vi "Flash Finish Stream.vi"(8 "error in (no error)":errorcluster, 11 "Orca-Flash 4.0 V2 in":refnum<class "Orca-Flash 4.0 V2.lvclass">) -> (0 "error out":errorcluster, 3 "Orca-Flash 4.0 V2 out":refnum<class "Orca-Flash 4.0 V2.lvclass">)   [LabVIEW 2017, in "Orca-Flash 4.0 V2.lvlib" / "Orca-Flash 4.0 V2.lvclass"]
uses:
  Orca-Flash 4.0 V2.lvclass
  C:/LVDEV/branch3/Flash Gordon v0.6.1b/Hardware/Camera/Camera.lvclass
  Orca-Flash 4.0 V2.lvclass/Orca-Flash 4.0 V2.ctl
  Resources/GLOBAL/GLOBAL Time-critical.vi
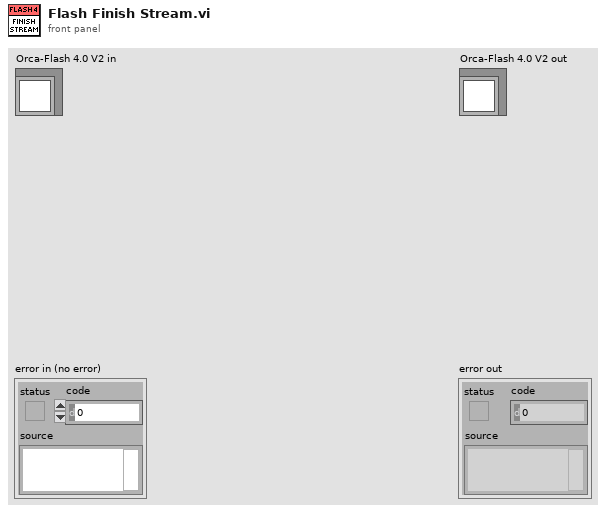
[diagram p1: front panel]
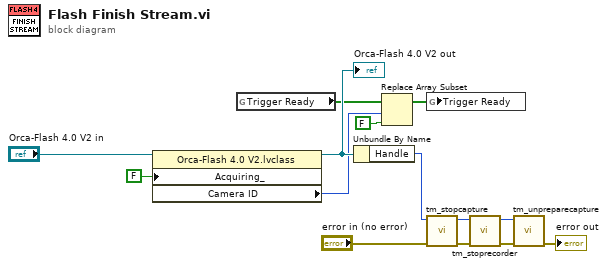
[diagram p0: block diagram]
diagram:
  n1 = property class="Orca-Flash 4.0 V2.lvclass"(reference="Orca-Flash 4.0 V2 in", "Acquiring_"=FALSE ("Live Mode")) -> (reference out=w11:refnum<class "Orca-Flash 4.0 V2.lvclass">, "Camera ID"=w4:i32)  [unwired: 1 in, 1 out]
  "Orca-Flash 4.0 V2 out" <- w11
  n2 = global read "GLOBAL Time-critical.vi" "Trigger Ready"() -> (w3:bool[])
  n3 = Unbundle By Name(w11) -> ("Handle"=w13:u32)
  n4 = Replace Array Subset(array=w3, new element=FALSE ("new element/subarray"), index=w4) -> (w2:bool[])
  n5 = global write "GLOBAL Time-critical.vi" "Trigger Ready"(w2) -> ()
  n6 = call <userlib>:"tm_stopcapture.vi"("error in (no error)"="error in (no error)", "Handle in"=w13) -> ("error out"=w8:errorcluster, "Handle out"=w5:u32)  [unwired: 8 in]
  n7 = call <userlib>:"tm_stoprecorder.vi"("error in (no error)"=w8, "Handle in"=w5) -> ("error out"=w7:errorcluster, "Handle out"=w6:u32)  [unwired: 8 in]
  n8 = call <userlib>:"tm_unpreparecapture.vi"("error in (no error)"=w7, "Handle in"=w6) -> ("error out"=→"error out":errorcluster)  [unwired: 8 in, 1 out]
